vi "Head-in-Head co-ord.vi"(1 "Velocity Vector (in space)":dbl[][](array[numeric]), 2 "Rotation Vector (in space)":dbl[][](array[numeric])) -> (0 "Velocity Vector (in coordinate frame)":dbl[][](array[numeric]))   [LabVIEW 2016]
uses:
  <vilib>/Analysis/baseanly.llb/Unit Vector (DBL).vi
  <vilib>/Analysis/baseanly.llb/Real Dot Product.vi
  fick-matrix/fick-matrix.lvlib
  <vilib>/Analysis/NI_AALBase.lvlib
panel:
  # "This VI will calculate the velocity of the object using the object as the frame of reference.\n\nFor example, given head-in-space position and velocity vectors this VI will output head-in-head velocity"
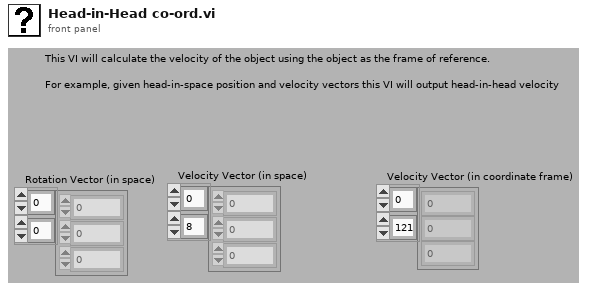
[diagram p1: front panel]
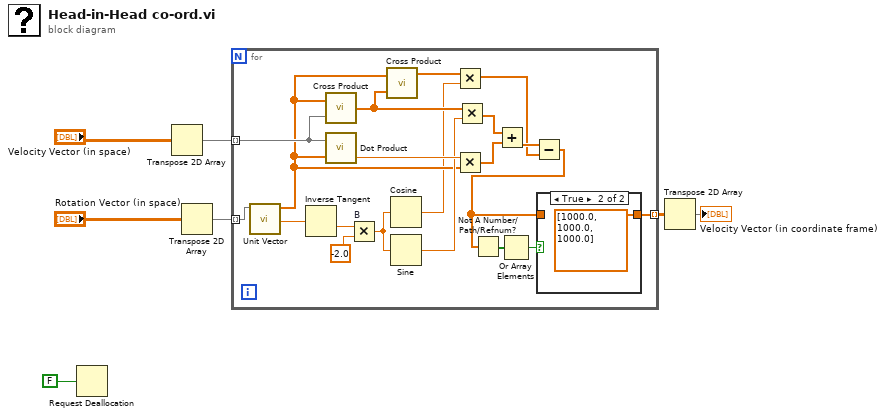
[diagram p0: block diagram]
diagram:
  n1 = Request Deallocation(FALSE ("flag")) -> ()
  n2 = Transpose 2D Array(2D array="Velocity Vector (in space)") -> (transposed array=w5:dbl[][])
  n3 = Transpose 2D Array(2D array="Rotation Vector (in space)") -> (transposed array=w4:dbl[][])
  n4 = for {
    tunnel: w4 -> [w27] mode=indexing
    tunnel: w5 -> [w21] mode=indexing
    tunnel: [w8] -> w3 mode=indexing
    n5 = call-poly <vilib>:"Unit Vector.vi"("Input Vector"=w27) -> ("norm"=w26:dbl, "Unit Vector"=w19:dbl[])  [unwired: 8 in, 1 out]
    n6 = Inverse Tangent(1:w26) -> (0:w25:dbl)
    n7 = call "Cross Product.vi"("B"=w21, "A"=w19) -> ("AxB"=w18:dbl[])
    n8 = call-poly <vilib>:"Dot Product.vi"("Y Vector"=w19, "X Vector"=w21) -> ("X * Y"=w22:dbl)  [unwired: 1 out]
    n9 = Multiply "B"(x=w25, y=-2.0) -> (x*y=w23:dbl)
    n10 = call "Cross Product.vi"("B"=w18, "A"=w19) -> ("AxB"=w16:dbl[])
    n11 = Cosine(x=w23) -> (cos(x)=w17:dbl)
    n12 = Sine(x=w23) -> (sin(x)=w20:dbl)
    n13 = Multiply ("B")(x=w16, y=w17) -> (x*y=w12:dbl[])
    n14 = Multiply ("B")(x=w22, y=w19) -> (x*y=w15:dbl[])
    n15 = Multiply ("B")(x=w18, y=w20) -> (x*y=w14:dbl[])
    n16 = Add(x=w14, y=w15) -> (x+y=w13:dbl[])
    n17 = Subtract(x=w13, y=w12) -> (x-y=w9:dbl[])
    n18 = Not A Number/Path/Refnum?(number/path/refnum=w9) -> (NaN/Path/Refnum?=w11:bool[])
    n19 = Or Array Elements(Boolean array=w11) -> (logical OR=w10:bool)
    n20 = case shown="True" w10 {
      tunnel: w9 -> [w28 _]
      tunnel: [w28 dbl[] [1000.0, 1000.0, 1000.0]] -> w8
      frame False {
      }
      frame True {
      }
    }
  }
  n21 = Transpose 2D Array(2D array=w3) -> (transposed array=→"Velocity Vector (in coordinate frame)":dbl[][])
